vi "Destroy.vi"(8 "error in (no error)":errorcluster, 11 "Stop Loop in":refnum<class "Stop Loop.lvclass">) -> (0 "error out":errorcluster)   [LabVIEW 2019, in "Test Executive.lvlib" / "Stop Loop.lvclass"]
uses:
  <vilib>/gpm_packages/@cs/test-executive/Source/Test Executive/Stop Loop/Stop Loop.lvclass
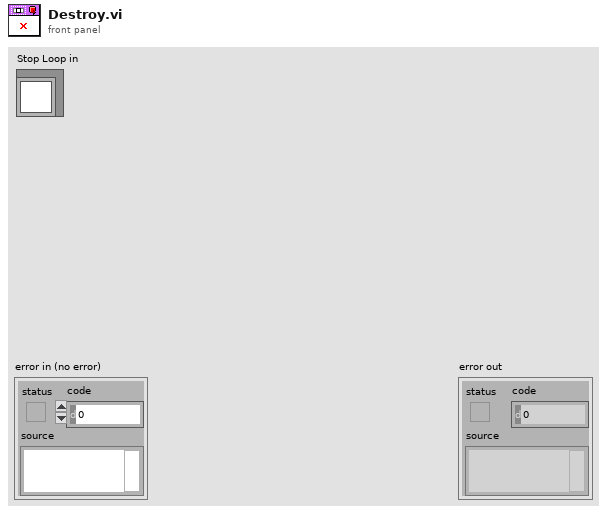
[diagram p1: front panel]
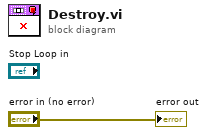
[diagram p0: block diagram]
diagram:
  "error out" <- "error in (no error)"
